vi "SetParameterInt.vi"(0 "Fehler (Eingang, kein Fehler)":errorcluster, 5 "instanceHandle":u32, 7 "DLL-Path":path, 9 "paramName":string, 11 "paramValue":i32) -> (4 "Fehler (Ausgang)":errorcluster, 6 "instanceHandle":u32, 8 "DLL-Path":path, 10 "ERR_CODE":i32)   [LabVIEW 2015, in "MEDAQLib.lvlib"]
doc: "ERR_CODE SetParameterInt (DWORD instanceHandle, LPCTSTR paramName, int paramValue);\n\nSet a 4 Byte integer parameter."
uses:
  MEDAQLib.lvlib
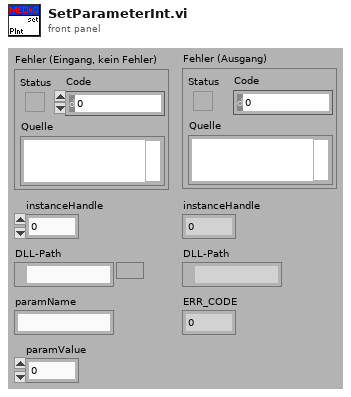
[diagram p1: front panel]
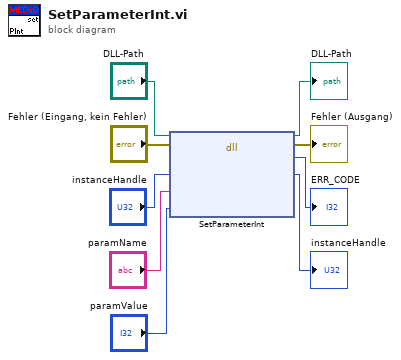
[diagram p0: block diagram]
diagram:
  n1 = dll-call lib="D:/Users/XRF/Desktop/Dante_acquire6/libs/Proximity_sensor/Release/MEDAQLib.dll" fn="SetParameterInt"(path in="DLL-Path", error in="Fehler (Eingang, kein Fehler)", "instanceHandle"="instanceHandle", "paramName"="paramName", "paramValue"="paramValue") -> (path out=→"DLL-Path":path, error out=→"Fehler (Ausgang)":errorcluster, "Rückgabetyp"=→"ERR_CODE":i32, "instanceHandle"=→"instanceHandle":u32)  [unwired: 3 in]
